vi "DMM SW Trigger.vi"(8 "error in (no error)":errorcluster, 11 "DMM in":refnum<class "NI DMM.lvclass">) -> (0 "error out":errorcluster, 3 "DMM out":refnum<class "NI DMM.lvclass">)   [LabVIEW 2020, in "NI DMM.lvlib" / "NI DMM.lvclass"]
uses:
  NI DMM.lvclass
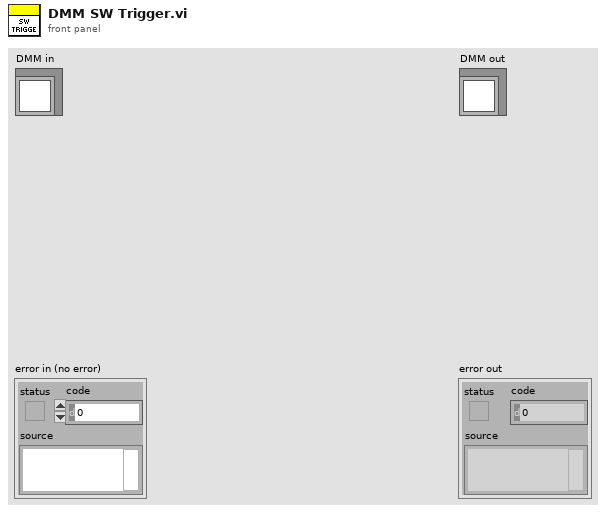
[diagram p1: front panel]
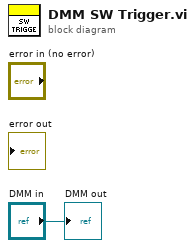
[diagram p0: block diagram]
diagram:
  "DMM out" <- "DMM in"
